vi "Debug.vi"(11 "Module in":refnum<class "Module.lvclass">) -> (2 "Debug":bool, 3 "Module out":refnum<class "Module.lvclass">)   [LabVIEW 2020, in "Volatus.lvlib" / "Module.lvclass"]
uses:
  Module.lvclass
  Module.lvclass/Module.ctl
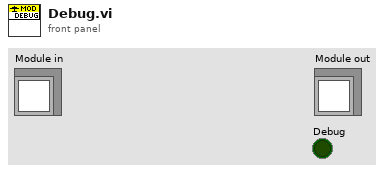
[diagram p1: front panel]
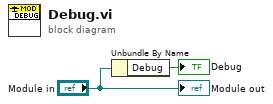
[diagram p0: block diagram]
diagram:
  n1 = Unbundle By Name("Module in") -> ("Debug"=→"Debug":bool)
  "Module out" <- "Module in"
